vi "Pascal Matrix_General.vi"(10 "columns":i32, 11 "rows":i32) -> (0 "error":i32, 3 "Pascal Matrix":dbl[][](array[numeric]))   [LabVIEW 2014, in "NI_AALPro.lvlib"]
uses:
  NI_AALPro.lvlib
  NI_Gmath.lvlib
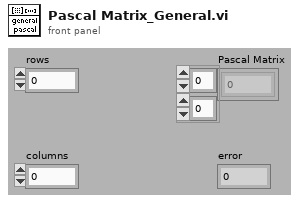
[diagram p1: front panel]
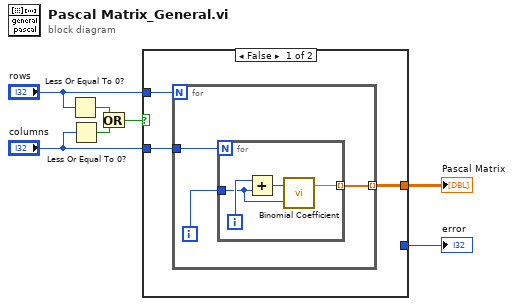
[diagram p0: block diagram]
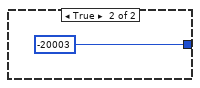
[diagram p2: hidden frame]
diagram:
  n1 = Less Or Equal To 0?(x="rows") -> (x <= 0?=w4:bool)
  n2 = Less Or Equal To 0?(x="columns") -> (x <= 0?=w3:bool)
  n3 = Or(x=w4, y=w3) -> (x .or. y?=w2:bool)
  n4 = case shown="False" w2 {
    tunnel: [w10 _] -> w7
    tunnel: "rows" -> [w9 _]
    tunnel: "columns" -> [w8 _]
    tunnel: [_ -20003] -> w1
    frame False {
      n5 = for {
        N: w9 -> [_]
        tunnel: w8 -> [w13]
        tunnel: [w11] -> w10 mode=indexing
        i -> [w12]
        n6 = for {
          N: w13 -> [_]
          tunnel: w12 -> [w15]
          tunnel: [w14] -> w11 mode=indexing
          i -> [w16]
          n7 = Add(x=w16, y=w15) -> (x+y=w17:i32)
          n8 = call "Binomial Coefficient.vi"("k"=w15, "n"=w17) -> ("binomial coefficient (n,k)"=w14:dbl)  [unwired: 1 out]
        }
      }
    }
    frame True {
    }
  }
  "Pascal Matrix" <- w7
  "error" <- w1
